vi "AR Drone - Gamepad Control.vi"() -> ()   [LabVIEW 2014]
doc: "Example demonstrating how to control the AR Drone with a joystick or gamepad."
uses:
  <vilib>/Utility/inputDevices.llb/closeJoystick.vi
  <vilib>/LVH/AR Drone Toolkit/AR Drone.lvlib
panel:
  out "Axes Output":T1 {"Vertical Speed" scale=-1.0..1.0; "Yaw Speed" scale=-1.0..1.0; "Pitch" scale=-1.0..1.0; "Roll" scale=-1.0..1.0}
  out "Gamepad Output":T2
  in  "stop":bool
  # "Xbox Controller:\nLeft stick L/R - Roll\nLeft stick D/U - Pitch\nL/R Triggers - Vertical Speed\nRight stick L/R - Yaw Speed"
  # "Xbox Controller:\nA - take off\nB - emergency\nX - hover\nStart - Stop"
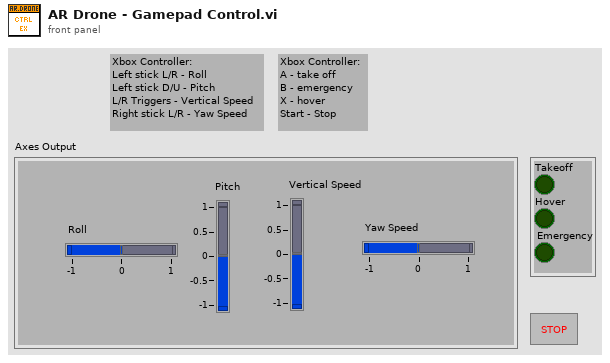
[diagram p1: front panel]
types:
  T1 = cluster{"Roll":dbl, "Pitch":dbl, "Vertical Speed":dbl, "Yaw Speed":dbl}
  T2 = cluster{"Takeoff":bool, "Hover":bool, "Emergency":bool, "Stop":bool, "Animation":bool}
  T3 = typedef "AR Drone.lvlib/AR Drone Resource.ctl" = cluster{"UDP Control Connection":refnum<k16>, "UDP NavData Connection":refnum<k16>, "UDP Video Connection (Drone 1.0)":refnum<k16>, "TCP Video Connection (Drone 2.0)":refnum<k5>, "TCP Control Port Connection":refnum<k5>, "Drone IP address":string, "Drone Command Port":u16, "Drone NavData Port":u16, "Drone Vid Stream Port":u16, "Drone TCP Control Port":u16, "Home IP address":string, "Home Command Port":u16, "Home NavData Port":u16, "Home Vid Stream Port":u16, "Drone Version":i32}
  T4 = cluster{"Roll":sgl, "Pitch":sgl, "Vertical Speed":sgl, "Yaw Speed":sgl}
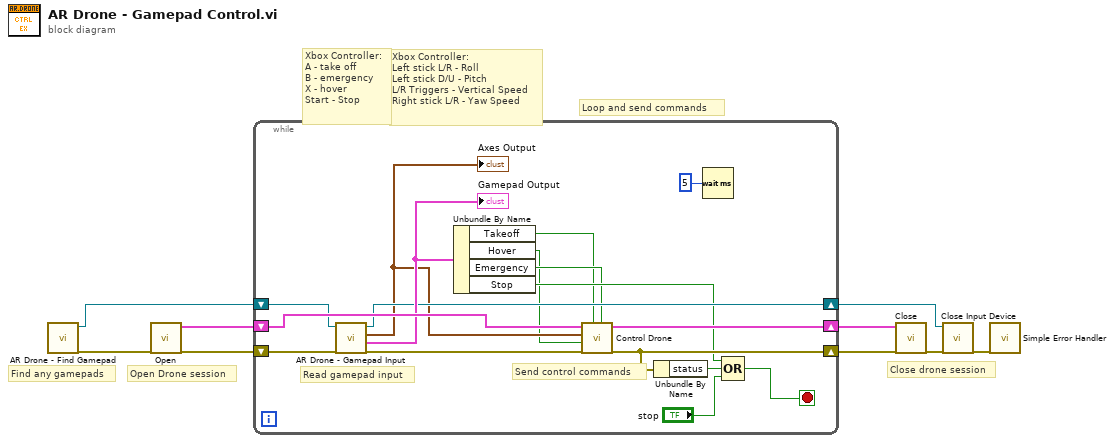
[diagram p0: block diagram]
diagram:
  # "Loop and send commands"
  # "Close drone session"
  # "Open Drone session"
  # "Find any gamepads"
  # "Xbox Controller:\nLeft stick L/R - Roll\nLeft stick D/U - Pitch\nL/R Triggers - Vertical Speed\nRight stick L/R - Yaw Speed"
  # "Xbox Controller:\nA - take off\nB - emergency\nX - hover\nStart - Stop"
  n1 = call "AR Drone - Find Gamepad.vi"() -> ("error out"=w1:errorcluster, "Refnum out"=w2:refnum<k1>)  [unwired: 10 in]
  n2 = call <vilib>:"Open.vi"("error in (no error)"=w1) -> ("error out"=w3:errorcluster, "AR Drone Resource"=w4:T3)  [unwired: 9 in]
  n3 = while {
    shift-right: [w25] -> w8
    shift-left: w4 -> [w26]
    shift-right: [w24] -> w9
    shift-left: w3 -> [w18]
    shift-right: [w15] -> w7
    shift-left: w2 -> [w19]
    stop <- w22 stop-if-true
    # "Send control commands"
    # "Read gamepad input"
    n4 = call "AR Drone - Gamepad Input.vi"("error in (no error)"=w18, "Refnum in"=w19) -> ("error out"=w17:errorcluster, "Gamepad Output"=w16:T2, "Control Cluster"=w14:T4, "Refnum out"=w15:refnum<k1>)  [unwired: 6 in]
    "Gamepad Output" <- w16
    "Axes Output" <- w14
    n5 = Unbundle By Name(w16) -> ("Takeoff"=w10:bool, "Hover"=w11:bool, "Emergency"=w12:bool, "Stop"=w13:bool)
    n6 = call <vilib>:"Control Drone.vi"("Emergency Landing"=w12, "Takeoff/Land"=w10, "error in (no error)"=w17, "Hover"=w11, "Control Cluster"=w14, "AR Drone Resource"=w26) -> ("error out"=w24:errorcluster, "AR Drone Resource Out"=w25:T3)  [unwired: 4 in]
    n7 = Unbundle By Name(w24) -> ("status"=w21:bool)
    n8 = Wait (ms)(milliseconds to wait=u32 5) -> ()  [unwired: 1 out]
    n9 = Compound Arithmetic op=OR(w13, w21, "stop") -> (w22:bool)
  }
  n10 = call <vilib>:"Close.vi"("error in (no error)"=w9, "AR Drone Resource"=w8) -> ("error out"=w6:errorcluster)  [unwired: 9 in]
  n11 = call-poly <vilib>:"Close Input Device.vi"("error in (no error)"=w6, "device ID"=w7) -> ("error out"=w5:errorcluster)  [unwired: 8 in]
  n12 = call <vilib>:"Simple Error Handler.vi"("error in (no error)"=w5) -> ()  [unwired: 4 in, 5 out]
